vi "dfd_Get FXP String Info from Type.vi"(7 "Include Overflow Status?":bool, 8 "error in (no error)":errorcluster, 11 "fxp type":T1={"Signed"=TRUE, "Word Length"=16, "Integer Word Length"=1}) -> (0 "error out":errorcluster, 3 "FXP Info String":string="fixed-point <±,16,1> [-1.000000E+0,9.999695E-1]:3.051758E-5")   [LabVIEW 2017, in "NI_DigFilterLicensed.lvlib"]
uses:
  <vilib>/addons/Digital Filter Design/NI_DigFilterLicensed.lvlib
  <vilib>/fxp/LVFixedPointRepBitsTypeDef.ctl
  <vilib>/Utility/VariantDataType/VariantType.lvlib
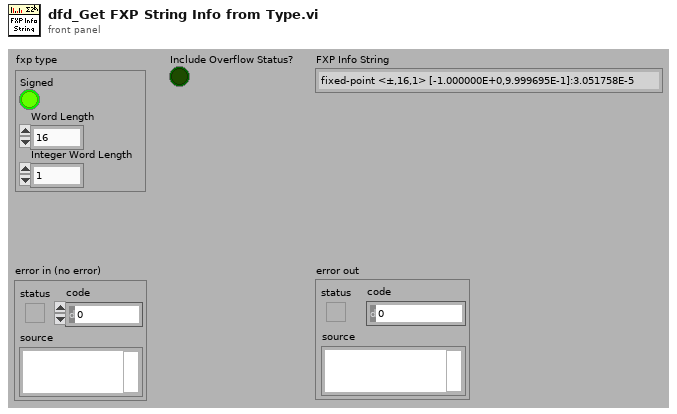
[diagram p1: front panel]
types:
  T1 = typedef "LVFixedPointRepBitsTypeDef.ctl" = cluster{"Signed":bool, "Word Length":u32, "Integer Word Length":i32}
  T2 = typedef "LVFixedPointRepRangeTypeDef.ctl" = cluster{"Range Min":dbl, "Range Max":dbl, "Delta":dbl}
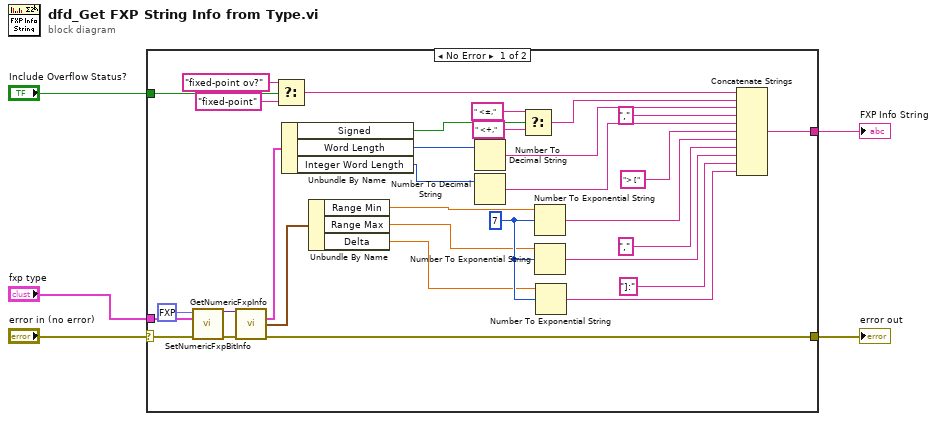
[diagram p0: block diagram]
diagram:
  n1 = case shown="No Error" "error in (no error)" {
    selector: "error in (no error)" -> [w33 w38]
    tunnel: "fxp type" -> [w34 _]
    tunnel: [w11 _] -> w2
    tunnel: [w10 w38] -> w3
    tunnel: "Include Overflow Status?" -> [w9 _]
    frame No Error {
      w20 = i16 7 ("width (-)")
      n2 = call <vilib>:"SetNumericFxpBitInfo.vi"("Variant"=fxp<+,1,1> 0.0, "FxpRepresentation"=w34, "error in (no error)"=w33) -> ("Modified Variant"=w37:variant, "error out"=w36:errorcluster)  [unwired: 11 out]
      n3 = call <vilib>:"GetNumericFxpInfo.vi"("Variant"=w37, "error in (no error)"=w36) -> ("FxpRepresentation"=w25:T1, "FxpRangeRepresentation"=w15:T2, "error out"=w10:errorcluster)  [unwired: 11 out]
      n4 = Select(t="fixed-point ov?" ("string"), s=w9, f="fixed-point" ("string")) -> (s? t:f=w6:string)
      n5 = Unbundle By Name(w25) -> ("Signed"=w24:bool, "Word Length"=w19:u32, "Integer Word Length"=w17:i32)
      n6 = Unbundle By Name(w15) -> ("Range Min"=w14:dbl, "Range Max"=w13:dbl, "Delta"=w12:dbl)
      n7 = Number To Decimal String(number=w19) -> (decimal integer string=w18:string)  [unwired: 1 out]
      n8 = Number To Decimal String(number=w17) -> (decimal integer string=w16:string)  [unwired: 1 out]
      n9 = Select(t=" <±," ("string"), s=w24, f=" <+," ("string")) -> (s? t:f=w21:string)
      n10 = Number To Exponential String(number=w14, 3:w20) -> (E-format string=w27:string)  [unwired: 2 out]
      n11 = Number To Exponential String(number=w13, 3:w20) -> (E-format string=w29:string)  [unwired: 2 out]
      n12 = Number To Exponential String(number=w12, 3:w20) -> (E-format string=w31:string)  [unwired: 2 out]
      n13 = Concatenate Strings(w6, w21, w18, "," ("string"), w16, "> [" ("string"), w27, "," ("string"), w29, "]:" ("string"), w31) -> (w11:string)
    }
    frame Error {
    }
  }
  "error out" <- w3
  "FXP Info String" <- w2
